vi "macro_Rotation3d_Axis_AngleRad.vi"   [LabVIEW 2019, in "Trajectory_Library.lvlib"]
uses:
  Util_CalcDist.vi
  Trajectory_Library.lvlib
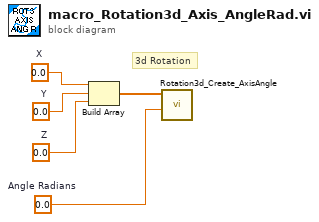
[diagram p0: block diagram]
diagram:
  w1 = 0.0  # Angle Radians
  w2 = 0.0  # Z
  w4 = 0.0  # X
  w3 = 0.0  # Y
  # "3d Rotation"
  n1 = Build Array(w4, w3, w2) -> (w5:dbl[])
  n2 = call "Rotation3d_Create_AxisAngle.vi"("Angle"=w1, "Axis Vector"=w5) -> ()  [unwired: 9 in, 1 out]
